vi "Error Message.vi"(8 "error in (no error)":errorcluster, 10 "error code":i32, 11 "SQL Statement In":refnum<class "SQL Statement.lvclass">) -> (0 "error out":errorcluster, 3 "SQL Statement Out":refnum<class "SQL Statement.lvclass">)   [LabVIEW 2023, in "SQLite.lvlib" / "SQL Statement.lvclass"]
uses:
  SQL Statement.lvclass
  SQLite.lvlib
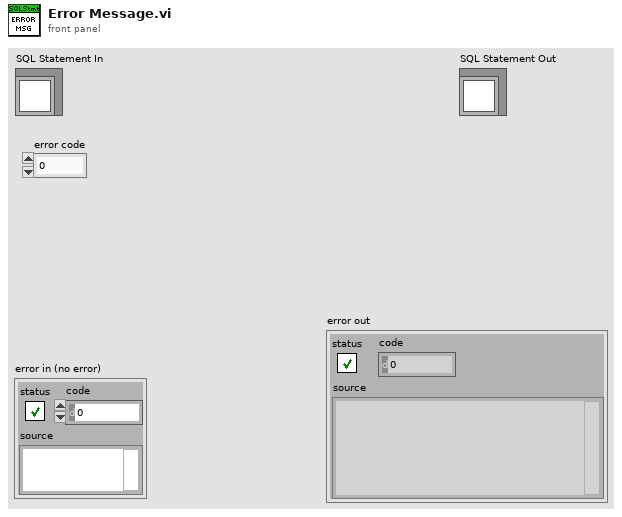
[diagram p1: front panel]
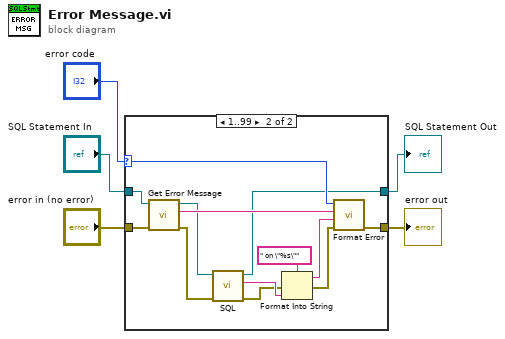
[diagram p0: block diagram]
diagram:
  n1 = case shown="1..99" "error code" {
    selector: "error code" -> [_ w17]
    tunnel: "SQL Statement In" -> [w6 w19]
    tunnel: "error in (no error)" -> [w7 w18]
    tunnel: [w7 w20] -> w3
    tunnel: [w6 w14] -> w1
    frame 0, Default {
    }
    frame 1..99 {
      n2 = call "Get Error Message.vi"("error in (no error)"=w18, "SQL Statement In"=w19) -> ("error out"=w13:errorcluster, "error message"=w16:string, "SQL Statement Out"=w15:refnum<class "SQL Statement.lvclass">)  [unwired: 7 in]
      n3 = call "SQL.vi"("error in (no error)"=w13, "SQL Statement in"=w15) -> ("error out"=w11:errorcluster, "SQL"=w12:string, "SQL Statement out"=w14:refnum<class "SQL Statement.lvclass">)  [unwired: 7 in]
      n4 = Format Into String(format string=" on \"%s\"", error in=w11, w12) -> (resulting string=w9:string, error out=w10:errorcluster)  [unwired: 1 in]
      n5 = call "Format Error.vi"("error in (no error)"=w10, "Additional source description"=w9, "error message"=w16, "error code"=w17) -> ("error out"=w20:errorcluster)  [unwired: 7 in]
    }
  }
  "error out" <- w3
  "SQL Statement Out" <- w1
